vi "13- Leading zeros SUBVI.vi"(11 "Input string":string) -> (3 "String":string)   [LabVIEW 2019]
panel:
  # "SUBVI TO REMOVE LEADING ZEROS FROM  STRING"
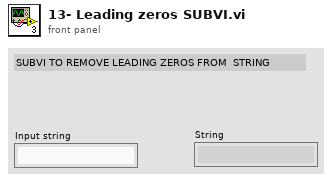
[diagram p1: front panel]
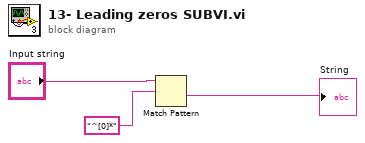
[diagram p0: block diagram]
diagram:
  n1 = Match Pattern(string="Input string", regular expression="^[0]*") -> (after substring=→"String":string)  [unwired: 1 in, 3 out]
